vi "rqcAlice Picture Demo (Low Level Example).vi"() -> ()   [LabVIEW 2019]
panel:
  in  "Corrected Alice's key path":string
  in  "Bob's port":string
  in  "Bob's IP":string
  out "pyton script path":path=path "../python_scripts/cascade_alice.py"
  in  "error in":errorcluster
  in  "path to PNG file":path
  out "?":picture
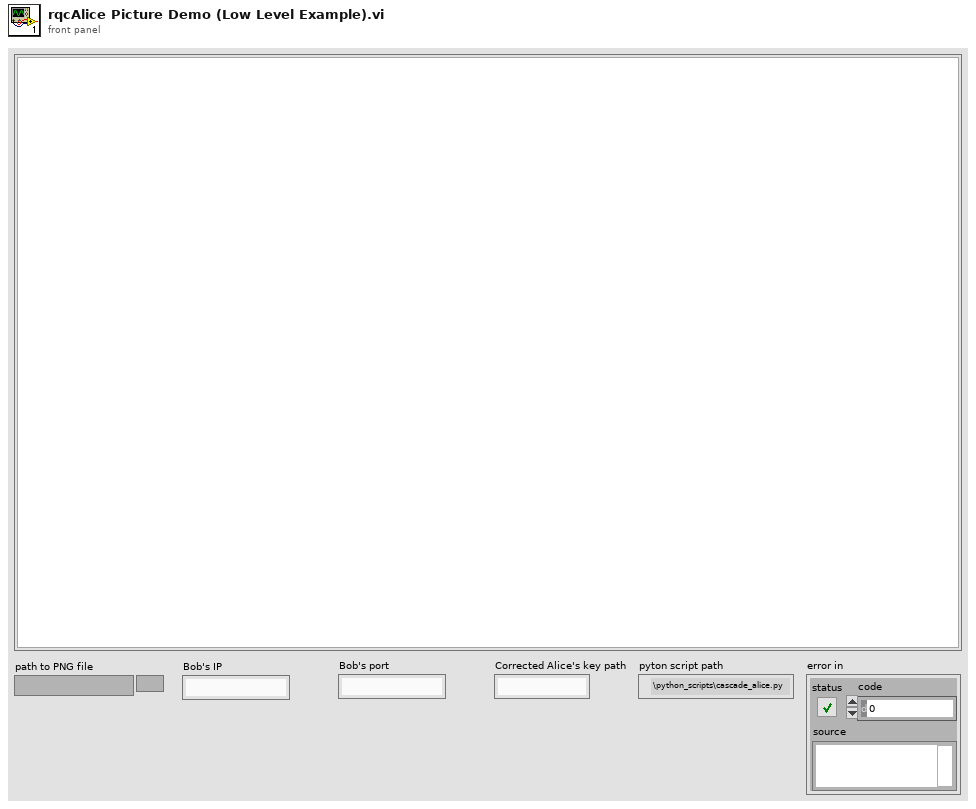
[diagram p1: front panel]
types:
  T1 = typedef "imagedata.ctl" = cluster{"image type":i32, "image depth":i32, "image":u8[], "mask":u8[], "colors":u32[], "Rectangle":cluster{"left":i16, "top":i16, "right":i16, "bottom":i16}}
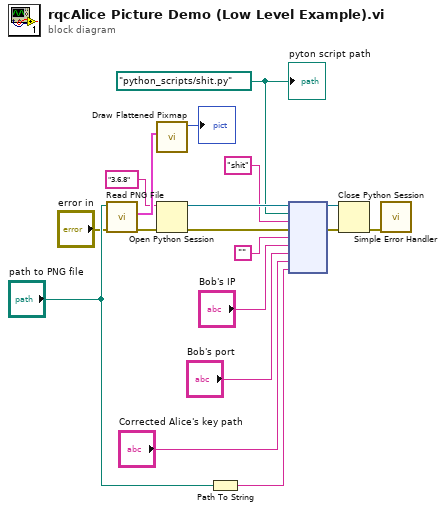
[diagram p0: block diagram]
diagram:
  w11 = path "python_scripts/shit.py" ("module path")
  n1 = call <vilib>:"Read PNG File.vi"("error in (no error)"="error in", "path to PNG file"="path to PNG file") -> ("error out"=w2:errorcluster, "image data"=w18:T1)  [unwired: 7 in, 1 out]
  n2 = call <vilib>:"Draw Flattened Pixmap.vi"("image data"=w18) -> ("new picture"=→"?":picture)  [unwired: 8 in]
  n3 = Open Python Session(python version="3.6.8" ("Python version"), 3:w2) -> (session out=w15:refnum<k35>, error out=w14:errorcluster)  [unwired: 1 in]
  n4 = Path To String(path="path to PNG file") -> (string=w4:string)
  n5 = node(w15, w11, "shit" ("function name"), w14, "", "Bob's IP", "Bob's port", "Corrected Alice's key path", w4) -> (w13:refnum<k35>, w6:errorcluster)  [unwired: 5 in, 2 out]
  n6 = Close Python Session(session in=w13, error in=w6) -> (11:w1:errorcluster)
  n7 = call <vilib>:"Simple Error Handler.vi"("error in (no error)"=w1) -> ()  [unwired: 4 in, 5 out]
  "pyton script path" <- w11
